vi "Delete Files.vi"(6 "Error Message in":string, 8 "Error In":errorcluster, 10 "Full App Name":string="PC Interface.exe", 11 "Server Files Cluster":T1) -> (0 "Error Out":errorcluster, 2 "Files Deleted":bool, 3 "Temp path Array":path[](array[path]), 4 "Error Message out":string)   [LabVIEW 2019]
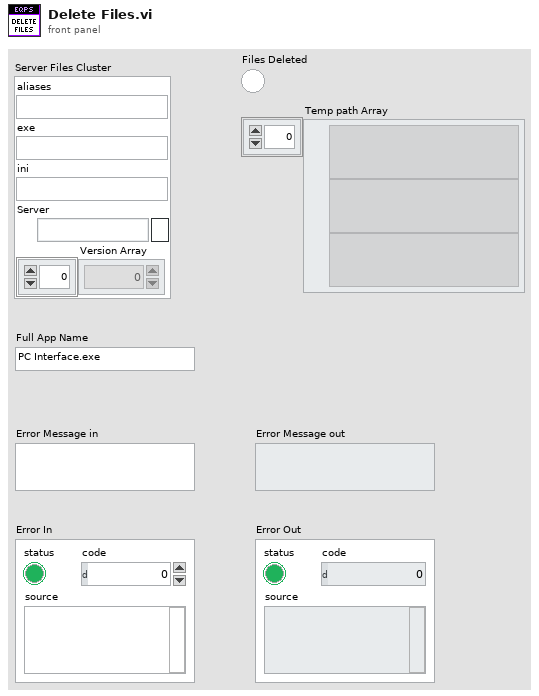
[diagram p1: front panel]
types:
  T1 = cluster{"aliases":string, "exe":string, "ini":string, "Server":path, "Version Array":i32[]}
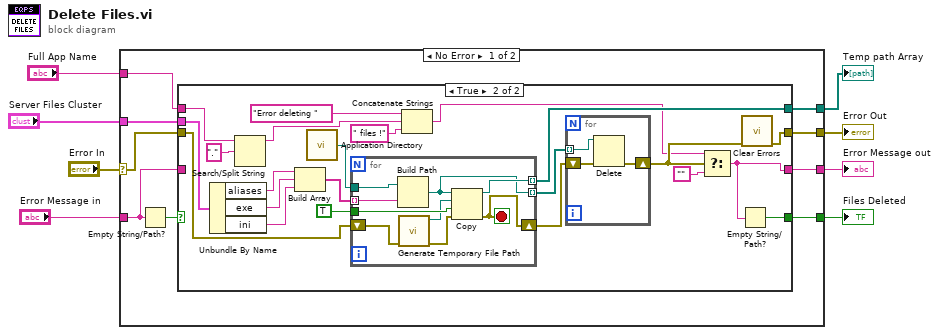
[diagram p0: block diagram]
diagram:
  n1 = case shown="No Error" "Error In" {
    selector: "Error In" -> [w13 w55]
    tunnel: [w14 w55] -> w7
    tunnel: [w16 w54] -> w6
    tunnel: "Error Message in" -> [w15 w54]
    tunnel: "Server Files Cluster" -> [w12 _]
    tunnel: [w11 _] -> w3
    tunnel: [w10 _] -> w2
    tunnel: "Full App Name" -> [w9 _]
    frame No Error {
      n2 = Empty String/Path?(string/path=w15) -> (empty?=w17:bool)
      n3 = case shown="True" w17 {
        tunnel: [w19 w27] -> w16
        tunnel: w15 -> [w19 _]
        tunnel: [w18 w29] -> w14
        tunnel: w13 -> [w18 w26]
        tunnel: w12 -> [_ w40]
        tunnel: [_ w33] -> w11
        tunnel: [_ w28] -> w10
        tunnel: w9 -> [_ w24]
        frame False {
        }
        frame True {
          n4 = Unbundle By Name(w40) -> ("aliases"=w37:string, "exe"=w39:string, "ini"=w38:string)
          n5 = Search/Split String(string=w24, search string/char (-)=".") -> (substring before match=w21:string)  [unwired: 1 in, 2 out]
          n6 = Build Array(w37, w39, w38) -> (w36:string[])
          n7 = call <vilib>:"Application Directory.vi"() -> ("Application Directory"=w41:path)
          n8 = for {
            tunnel: w41 -> [w53]
            tunnel: w36 -> [w52] mode=indexing
            shift-right: [w45] -> w32
            shift-left: w26 -> [w47]
            tunnel: TRUE ("overwrite (F)") -> [w51]
            tunnel: [w50] -> w33 mode=indexing
            tunnel: [w49] -> w34 mode=indexing
            stop <- w45 stop-if-true
            n9 = Build Path(base path=w53, name or relative path=w52) -> (appended path=w49:path)
            n10 = call <vilib>:"Generate Temporary File Path.vi"("error in (no error)"=w47) -> ("error out"=w46:errorcluster, "Unique Temporary File Path"=w48:path)  [unwired: 9 in]
            n11 = Copy(8:w46, 9:w51, 10:w48, 11:w49) -> (0:w45:errorcluster, 3:w50:path)  [unwired: 1 in, 1 out]
          }
          n12 = Concatenate Strings("Error deleting ", w21, " files !") -> (w23:string)
          n13 = for {
            tunnel: w34 -> [w42] mode=indexing
            shift-right: [w43] -> w31
            shift-left: w32 -> [w44]
            n14 = Delete(path (use dialog)=w42, error in=w44) -> (error out=w43:errorcluster)  [unwired: 3 in, 2 out]
          }
          n15 = Select(t=w23, s=w31, f="") -> (s? t:f=w27:string)
          n16 = Empty String/Path?(string/path=w27) -> (empty?=w28:bool)
          n17 = call <vilib>:"Clear Errors.vi"("error in (no error)"=w31) -> ("error out"=w29:errorcluster)  [unwired: 5 in, 1 out]
        }
      }
    }
    frame Error {
    }
  }
  "Error Out" <- w7
  "Error Message out" <- w6
  "Files Deleted" <- w2
  "Temp path Array" <- w3
